vi "Dashboard Main.vi"() -> ()   [LabVIEW 2012]
uses:
  <vilib>/event_ctls.llb/eventvkey.ctl
  <vilib>/Utility/miscctls.llb/LVPointTypeDef.ctl
  <vilib>/Utility/config.llb/Read Key (String).vi
  <vilib>/Utility/config.llb/Read Key (I32).vi
  <vilib>/Utility/config.llb/Write Key (String).vi
  <vilib>/Utility/config.llb/Write Key (I32).vi
  <vilib>/Utility/config.llb/NI_LVConfig.lvlib
panel:
  out "Battery Value":dbl(slide) scale=0.0..14.0 scale format="%#_2e"
  out "Battery":sgl(graph)
  in  "Camera Settings":T1={"Frate Rate"=30, "Compression"=30, "Size"=0} {"Frate Rate" scale=1.0..30.0; "Size" items=["640x480", "320x240", "160x120"]}
  out "Mode":T2(ring)=enum.""
  out "Camera IP":string="10.16.76.11"
  out "JS1 Z":dbl(slide) scale=-1.0..1.0 scale format="%#_2e"
  out "JS2 Z":dbl(slide) scale=-1.0..1.0 scale format="%#_2e"
  out "Joystick 1":cluster{"X":dbl, "Y":dbl}[](graph)
  out "Joystick 2":cluster{"X":dbl, "Y":dbl}[](graph)
  out "JS Buttons 1":T3
  out "JS Buttons 2":T3
  out "MotorSlide4":dbl(slide) scale=-1.0..1.0 scale format="%#_2e"
  out "MotorSlide3":dbl(slide) scale=-1.0..1.0 scale format="%#_2e"
  out "MotorSlide2":dbl(slide) scale=-1.0..1.0 scale format="%#_2e"
  in  "MotorName3":string="Front Left"
  in  "MotorName4":string="Front Right"
  in  "MotorName1":string="Rear Left"
  in  "MotorName2":string="Rear Right"
  out "MotorChart4":dbl(graph)
  out "MotorChart3":dbl(graph)
  out "MotorChart2":dbl(graph)
  out "MotorSlide1":dbl(slide) scale=-1.0..1.0 scale format="%#_2e"
  out "MotorChart1":dbl(graph)
  out "Robot IP":string="0.0.0.0"
  in  "Dashboard Tab":enum32{"Operation", "Test", "Checklist"}(tab)
  out "Dashboard Code Verzion":string
  out "Robot Code Verzion":string
  out "Gyro":dbl
  out "Encoder Average":dbl
  out "Right Encoder":dbl
  out "Left Encoder":dbl
  out "Vision Angle":dbl
  in  "Slider":dbl(slide) scale=0.0..100.0 scale format="%#_3g"
  in  "On/Off":bool caption="Solenoid"
  in  "Test Name":u16(ring) items=["Select the test to run...", "Example Test", "-------------------------------", "List of tests is built in robot code.", "Replace with your own automated tests."]
  in  "Test Tree":string(tree)
  in  "Motor":cluster{"Value":dbl, "Enable":bool} {"Value" scale=-1.0..1.0 scale format="%#_3g"}
  out "Progress":T4 {"Test Progress" scale=0.0..100.0}
  in  "Rev/Fwd":cluster{"Forward":bool, "Reverse":bool}
  in  "Ring":u16(ring) items=["Auto", "Fixed indoor", "Fixed outdoor 1", "Fixed outdoor 2", "Fixed fluorescent 1", "Fixed fluorescent 2", "Hold current"]
  in  "Listbox":i32(listbox)
  in  "Viewer":T5(tab)
  out "Mbps":dbl format="%#.1g"
  in  "Enable":bool=TRUE
  in  "DB Camera Config":bool
  out "Mbps":bool
  out "fps":dbl format="%#.1g"
  out "Image Error Message":string="Timeout in Camera Communications"
  out "Camera Image":T6(plugin-control)
  out "Buttons 1":cluster{"1":bool, "2":bool, "3":bool}
  out "Kinect 1":cluster{"X":dbl, "Y":dbl, "Z":dbl} {"X" scale=1.0..-1.0; "Y" scale=1.0..-1.0; "Z" scale=1.0..-1.0}
  out "Buttons 2":cluster{"1":bool, "2":bool, "3":bool}
  out "Kinect 2":cluster{"X":dbl, "Y":dbl, "Z":dbl} {"X" scale=1.0..-1.0; "Y" scale=1.0..-1.0; "Z" scale=1.0..-1.0}
  out "Version":string
  out "Skeleton Picture":picture
  out "Players":i8
  out "Tree":string(tree)
  # "Drive & Motors"
  # "Robot IP:"
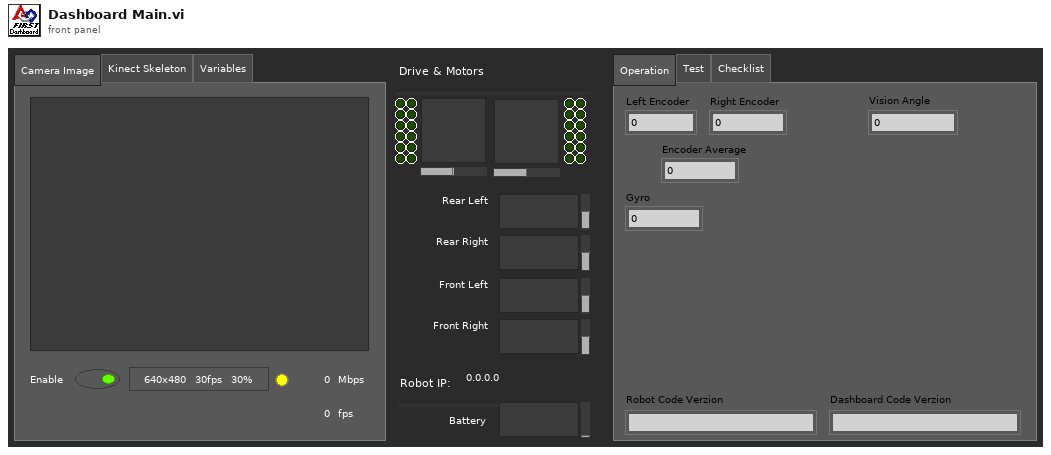
[diagram p1: front panel]
types:
  T1 = cluster{"Frate Rate":i32, "Compression":i32, "Size":u16}
  T2 = enum8{"Tele-Op Disabled", "Tele-Op Enabled", "Auto Disabled", "Auto Enabled", "Test Disabled", "Test Enabled", ""}
  T3 = cluster{bool, bool, bool, bool, bool, bool, bool, bool, bool, bool, bool, bool}
  T4 = cluster{"Test Progress":u8, "Test Progress Text":string}
  T5 = enum32{"Camera Image", "Kinect Skeleton", "Variables"}
  T6 = typedef "IMAQ Image.ctl" = refnum<image>
  T7 = typedef "Image Type" = u32
  T8 = cluster{"Competition mode":bool, "Robot Link":bool, "Autonomous":bool, "Enabled":bool, "E-Stop":bool, "Simulated":bool, "TestMode":bool, "Docked Window":bool}
  T9 = cluster{"Boolean Array[0]":bool, "Boolean Array[1]":bool, "Boolean Array[2]":bool, "Boolean Array[3]":bool, "Boolean Array[4]":bool, "Boolean Array[5]":bool, "Boolean Array[6]":bool, "Boolean Array[7]":bool, "Boolean Array[8]":bool, "Boolean Array[9]":bool, "Boolean Array[10]":bool, "Boolean Array[11]":bool}
  T10 = typedef "LVPointTypeDef.ctl" = cluster{"Horizontal":i16, "Vertical":i16}
  T11 = typedef "LVRectTypeDef.ctl" = cluster{"Left":i16, "Top":i16, "Right":i16, "Bottom":i16}
  T12 = typedef "LVBoundsTypeDef.ctl" = cluster{"Width":u32, "Height":u32}
  T13 = typedef "SkeletonTrackState.ctl" = enum32{"NotTracked", "PositionOnly", "Tracked"}
  T14 = cluster{"TrackingState":u8[], "Position":cluster{"x":sgl, "y":sgl, "z":sgl}, cluster{"x":sgl, "y":sgl, "z":sgl, sgl}[], "TrackState":T13}
  T15 = cluster{cluster{"ScaledToPercentRange":dbl, "ScaledToPercentRange":dbl, "ScaledToPercentRange":dbl}, cluster{bool, bool, bool}}[]
  T16 = cluster{cluster{"ScaledToPercentRange":dbl, "ScaledToPercentRange":dbl, "ScaledToPercentRange":dbl}, cluster{bool, bool, bool}}
  T17 = cluster{"ScaledToPercentRange":dbl, "ScaledToPercentRange":dbl, "ScaledToPercentRange":dbl}
  T18 = typedef "NI_LVConfig.lvlib/Config Data RefNum.ctl" = refnum<k1>
  T19 = typedef "eventvkey.ctl" = enum16{"ASCII", "Enter", "Return", "Shift", "Ctrl", "Alt", "Cmd", "Opt", "Caps", "NumLock", "Clear", "Break", "Up", "Down", "Left", "Right", "Insert", "Delete", "Home", "End", "PageUp", "PageDown", "Escape", "Help", "Pause", "ScrollLock", "F1", "F2", "F3", "F4", "F5", "F6", "F7", "F8", "F9", "F10", "F11", "F12", "F13", "F14", "F15", "F16", "F17", "F18", "F19", "F20", "F21", "F22", "F23", "F24", "Play", "VolumeUp", "VolumeDown", "Mute", "Two Byte Char"}
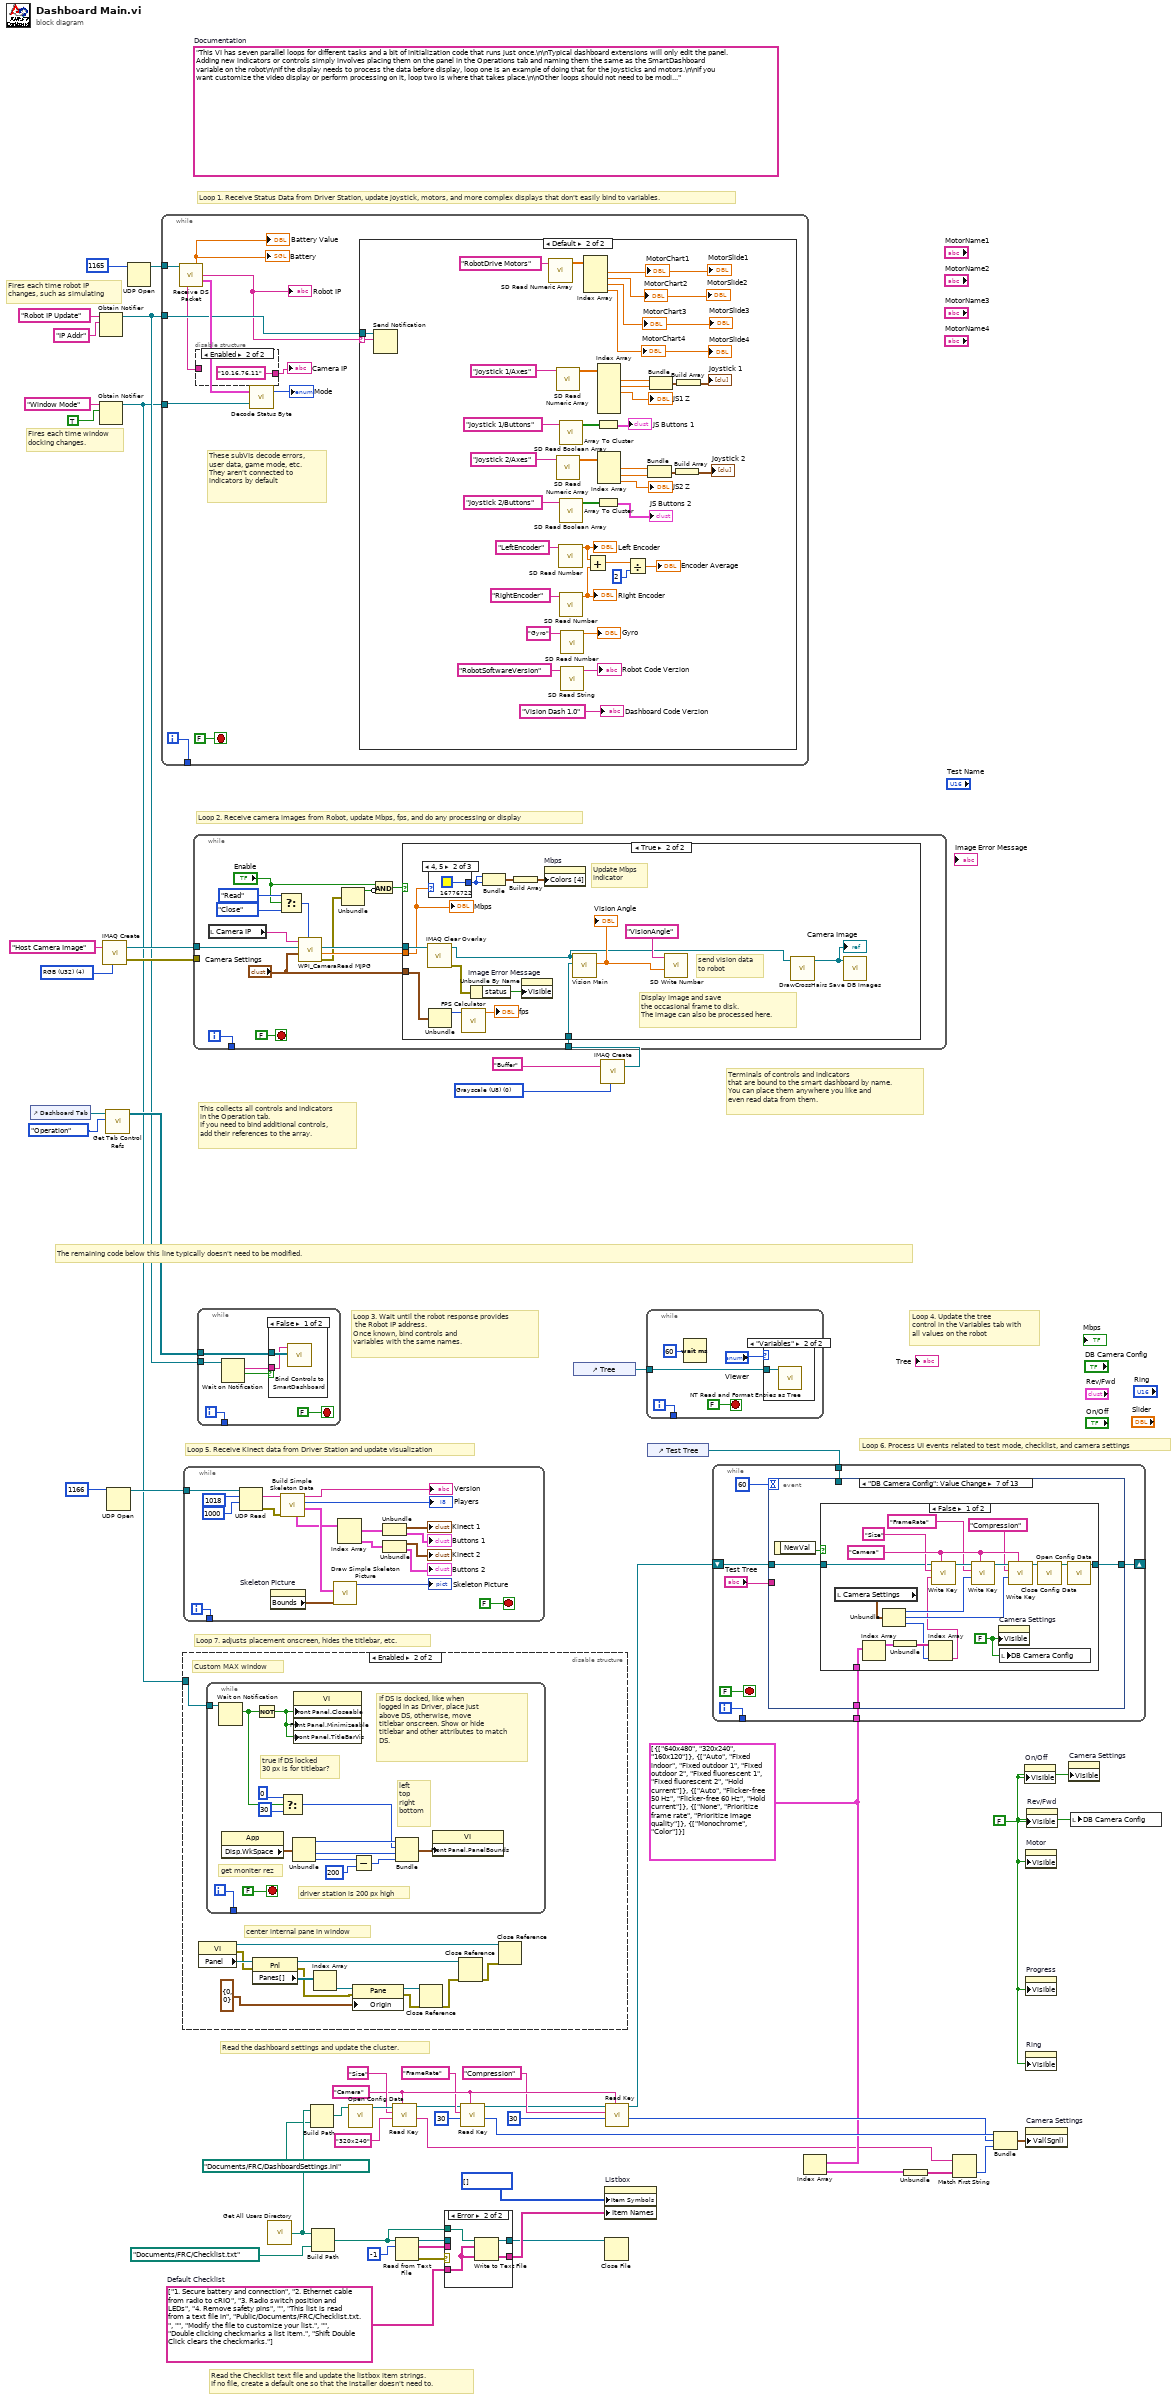
[diagram p0: block diagram]
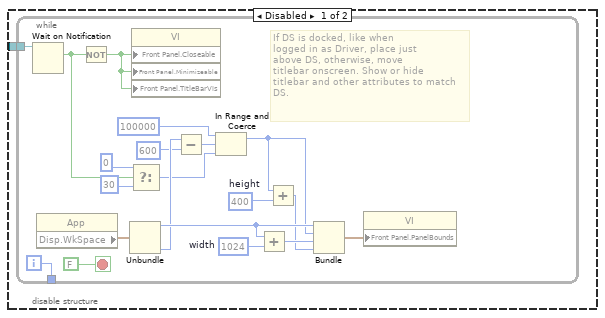
[diagram p2: hidden frame]
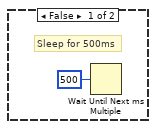
[diagram p4: hidden frame]
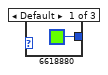
[diagram p5: hidden frame]
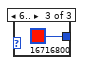
[diagram p6: hidden frame]
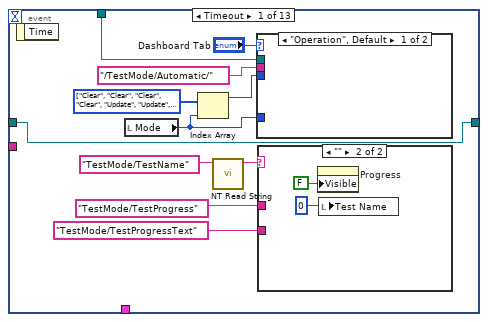
[diagram p8: hidden frame]
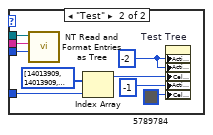
[diagram p9: hidden frame]
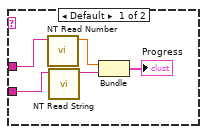
[diagram p10: hidden frame]
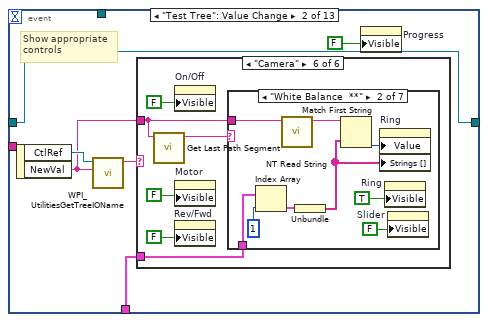
[diagram p11: hidden frame]
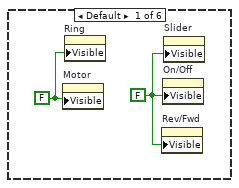
[diagram p12: hidden frame]
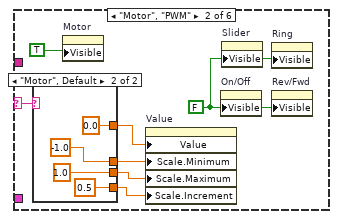
[diagram p13: hidden frame]
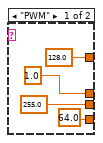
[diagram p14: hidden frame]
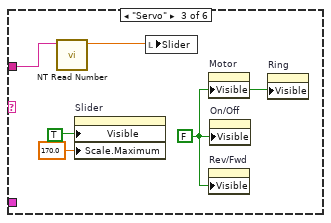
[diagram p15: hidden frame]
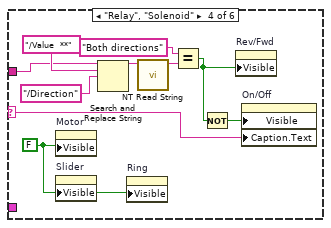
[diagram p16: hidden frame]
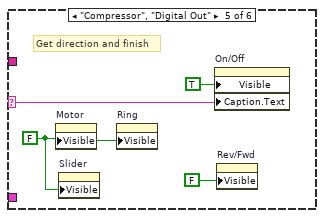
[diagram p17: hidden frame]
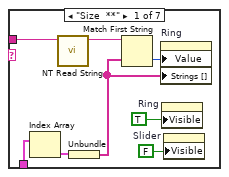
[diagram p18: hidden frame]
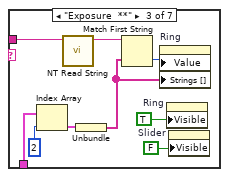
[diagram p19: hidden frame]
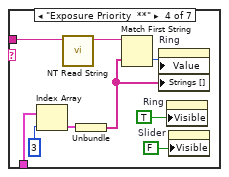
[diagram p20: hidden frame]
diagram:
  w2 = T7 0 items=["Grayscale (U8)", "Grayscale (I16)", "Grayscale (SGL)", "Complex (CSG)", "RGB (U32)", "HSL (U32)", "RGB (U64)", "Grayscale (U16)"] ("Image Type")
  w24 = "Camera"
  w16 = cluster{string[]}[] [{["640x480", "320x240", "160x120"]}, {["Auto", "Fixed indoor", "Fixed outdoor 1", "Fixed outdoor 2", "Fixed fluorescent 1", "Fixed fluorescent 2", "Hold current"]}, {["Auto", "Flicker-free 50 Hz", "Flicker-free 60 Hz", "Hold current"]}, {["None", "Prioritize frame rate", "Prioritize image quality"]}, {["Monochrome", "Color"]}]
  w32 = string[] ["1. Secure battery and connection", "2. Ethernet cable from radio to cRIO", "3. Radio switch position and LEDs", "4. Remove safety pins", "", "This list is read from a text file in", "Public/Documents/FRC/Checklist.txt.", "", "Modify the file to customize your list.", "", "Double clicking checkmarks a list item.", "Shift Double Click clears the checkmarks."]  # Default Checklist
  w30 = FALSE ("Visible")
  (unwired) "This VI has seven parallel loops for different tasks and a bit of initialization code that runs just once.\n\nTypical dashboard extensions will only edit the panel. Adding new indicators or controls simply involves placing them on the panel in the Operations tab and naming them the same as the SmartDashboard variable on the robot\n\nIf the display needs to process the data before display, loop one is an example of doing that for the joysticks and motors.\n\nIf you want customize the video display or perform processing on it, loop two is where that takes place.\n\nOther loops should not need to be modified. They are pretty standard, and document the task they perform."  # Documentation
  w53 = T7 4 items=["Grayscale (U8)", "Grayscale (I16)", "Grayscale (SGL)", "Complex (CSG)", "RGB (U32)", "HSL (U32)", "RGB (U64)"] ("Image Type")
  # "Fires each time robot IP\nchanges, such as simulating"
  # "Fires each time window\ndocking changes."
  # "Read the Checklist text file and update the listbox item strings.\nIf no file, create a default one so that the installer doesn't need to."
  # "This collects all controls and indicators\nin the Operation tab.\nIf you need to bind additional controls,\nadd their references to the array."
  # "The remaining code below this line typically doesn't need to be modified."
  # "Loop 6. Process UI events related to test mode, checklist, and camera settings"
  # "Read the dashboard settings and update the cluster."
  # "Terminals of controls and indicators\nthat are bound to the smart dashboard by name.\nYou can place them anywhere you like and\neven read data from them."
  # "Loop 4. Update the tree\ncontrol in the Variables tab with\nall values on the robot"
  # "Loop 3. Wait until the robot response provides\n the Robot IP address.\nOnce known, bind controls and\nvariables with the same names."
  # "Loop 5. Receive Kinect data from Driver Station and update visualization"
  # "Loop 7. adjusts placement onscreen, hides the titlebar, etc."
  # "Loop 1. Receive Status Data from Driver Station, update joystick, motors, and more complex displays that don't easily bind to variables."
  # "Loop 2. Receive camera images from Robot, update Mbps, fps, and do any processing or display"
  n1 = control-ref of="Dashboard Tab"() -> (w46:refnum<vi>)
  n2 = Obtain Notifier(name (unnamed)="Robot IP Update", notification data type="IP Addr" ("name (unnamed)")) -> (notifier out=w43:refnum<notifier>)  [unwired: 2 in, 2 out]
  n3 = Obtain Notifier(name (unnamed)="Window Mode", notification data type=TRUE) -> (notifier out=w36:refnum<notifier>)  [unwired: 2 in, 2 out]
  n4 = call "IMAQ Create"("Image Name"="Host Camera Image", "Image Type"=w53) -> ("New Image"=w51:T6, "error out"=w50:errorcluster)  [unwired: 2 in, 1 out]
  n5 = call <vilib>:"Get Tab Control Refs.vi"("Page Index"=enum32{"Operation", "Test"}."Operation" ("Dashboard Tab"), "TabControl in"=w46) -> ("ControlsOnPage"=w47:refnum<vi>[])  [unwired: 9 in]
  n6 = UDP Open(11:u16 1166 ("port")) -> (port=w48:refnum<k16>)  [unwired: 2 in, 4 out]
  n7 = UDP Open(11:u16 1165 ("port")) -> (port=w54:refnum<k16>)  [unwired: 2 in, 4 out]
  n8 = while {
    tunnel: w54 -> [w64]
    tunnel: w43 -> [w59]
    tunnel: w36 -> [w62]
    tunnel: [w60] -> _
    i -> [w60]
    stop <- FALSE stop-if-true
    # "These subVIs decode errors, user data, game mode, etc.\nThey aren't connected to indicators by default"
    n9 = call "Receive DS Packet.vi"("Recv Socket"=w64) -> ("Battery"=→"Battery" →"Battery Value":sgl, "Robot IP Address"=w58:string, "Status"=w65:T8, "Camera IP Address"=w56:string)  [unwired: 1 in, 10 out]
    "Robot IP" <- w58
    n10 = disable-structure shown="Enabled" {
      disable-tunnel: [w67 "10.16.76.11" ("Camera IP")] -> w57
      disable-tunnel: w56 -> [w67 _]
      frame Disabled {
      }
      frame Enabled {
      }
    }
    "Camera IP" <- w57
    n11 = call "Decode Status Byte.vi"("Window Mode Notifier"=w62, "Status"=w65) -> ("Mode"=→"Mode":T2)  [unwired: 1 out]
    n12 = case shown="Default" w58 {
      selector: w58 -> [_ w81]
      tunnel: w59 -> [_ w82]
      frame "0.0.0.0" {
        # "Robot not responding, don't poll the variables"
      }
      frame Default {
        n13 = Send Notification(notification=w81, notifier=w82) -> ()  [unwired: 1 in, 2 out]
        n14 = call <vilib>:"SD Read Numeric Array.vi"("Name"="RobotDrive Motors") -> ("Numeric Array"=w105:dbl[])  [unwired: 8 in, 2 out]
        n15 = call <vilib>:"SD Read Numeric Array.vi"("Name"="Joystick 1/Axes") -> ("Numeric Array"=w98:dbl[])  [unwired: 8 in, 2 out]
        n16 = call <vilib>:"SD Read Numeric Array.vi"("Name"="Joystick 2/Axes") -> ("Numeric Array"=w92:dbl[])  [unwired: 8 in, 2 out]
        n17 = call <vilib>:"SD Read Number.vi"("Name"="LeftEncoder") -> ("Numeric"=w77:dbl)  [unwired: 8 in, 2 out]
        "Left Encoder" <- w77
        n18 = call <vilib>:"SD Read Boolean Array.vi"("Name"="Joystick 1/Buttons") -> ("Boolean Array"=w100:bool[])  [unwired: 8 in, 2 out]
        n19 = call <vilib>:"SD Read Boolean Array.vi"("Name"="Joystick 2/Buttons") -> ("Boolean Array"=w91:bool[])  [unwired: 8 in, 2 out]
        n20 = call <vilib>:"SD Read Number.vi"("Name"="RightEncoder") -> ("Numeric"=w76:dbl)  [unwired: 8 in, 2 out]
        "Right Encoder" <- w76
        n21 = call <vilib>:"SD Read Number.vi"("Name"="Gyro") -> ("Numeric"=→"Gyro":dbl)  [unwired: 8 in, 2 out]
        n22 = call <vilib>:"SD Read String.vi"("Name"="RobotSoftwareVersion") -> ("String"=→"Robot Code Verzion":string)  [unwired: 8 in, 2 out]
        n23 = Index Array(array=w105) -> (element #1=→"MotorChart1" →"MotorSlide1":dbl, element #2=→"MotorSlide2" →"MotorChart2":dbl, element #3=→"MotorChart3" →"MotorSlide3":dbl, element #4=→"MotorChart4" →"MotorSlide4":dbl)  [unwired: 4 in]
        n24 = Add(x=w77, y=w76) -> (x+y=w74:dbl)
        n25 = Array To Cluster(array=w100) -> (cluster=→"JS Buttons 1":T9)
        n26 = Array To Cluster(array=w91) -> (cluster=→"JS Buttons 2":T9)
        n27 = Index Array(array=w98) -> (element #1=w95:dbl, element #2=w96:dbl, element #3=→"JS1 Z":dbl)  [unwired: 6 in, 3 out]
        n28 = Index Array(array=w92) -> (element #1=w87:dbl, element #2=w86:dbl, element #3=→"JS2 Z":dbl)  [unwired: 3 in]
        n29 = Divide(x=w74, y=2) -> (x/y=→"Encoder Average":dbl)
        n30 = Bundle("Numeric"=w87, "Numeric"=w86) -> (w88:cluster{"Numeric":dbl, "Numeric":dbl})  [unwired: 1 in]
        n31 = Bundle("Numeric"=w95, "Numeric"=w96) -> (w94:cluster{"Numeric":dbl, "Numeric":dbl})  [unwired: 1 in]
        n32 = Build Array(w88) -> (→"Joystick 2":cluster{"Numeric":dbl, "Numeric":dbl}[])
        n33 = Build Array(w94) -> (→"Joystick 1":cluster{"Numeric":dbl, "Numeric":dbl}[])
        "Dashboard Code Verzion" <- "Vision Dash 1.0" ("Dashboard Code Verzion")
      }
    }
  }
  n34 = disable-structure shown="Enabled" {
    disable-tunnel: w36 -> [w109 w142]
    frame Disabled {
      n35 = while {
        tunnel: w109 -> [w128]
        tunnel: [w126] -> _
        i -> [w126]
        stop <- FALSE stop-if-true
        w118 = 1024  # width
        w121 = 400  # height
        # "If DS is docked, like when\nlogged in as Driver, place just\nabove DS, otherwise, move\ntitlebar onscreen. Show or hide\ntitlebar and other attributes to match\nDS."
        n36 = Wait on Notification(notifier=w128) -> (notification=w113:bool)  [unwired: 3 in, 3 out]
        n37 = property class="App"() -> ("Disp.WkSpace"=w124:T11)  [unwired: 2 in, 2 out]
        n38 = Not(x=w113) -> (.not. x?=w127:bool)
        n39 = Unbundle(w124) -> ("Left"=w122:i16, "Bottom"=w119:i16)  [unwired: 2 out]
        n40 = Select(t=0, s=w113, f=30) -> (s? t:f=w112:i32)
        n41 = property class="VI"("Front Panel.Closeable"=w127, "Front Panel.Minimizeable"=w127, "Front Panel.TitleBarVis"=w127) -> ()  [unwired: 2 in, 2 out]
        n42 = Subtract(x=w119, y=600) -> (x-y=w116:i32)
        n43 = In Range and Coerce(upper limit=100000, x=w116, lower limit=w112) -> (coerced(x)=w110:i32)  [unwired: 1 out]
        n44 = Add(x=w122, y=w118) -> (x+y=w123:i32)
        n45 = Add(x=w110, y=w121) -> (x+y=w120:i32)
        n46 = Bundle("Left"=w122, w110, w123, w120) -> (w125:cluster{"Left":i16, i32, i32, i32})  [unwired: 1 out]
        n47 = property class="VI"("Front Panel.PanelBounds"=w125) -> ()  [unwired: 2 in, 2 out]
      }
    }
    frame Enabled {
      # "center internal pane in window"
      # "Custom MAX window"
      n48 = property class="VI"() -> (reference out=w135:refnum<vi>, error out=w134:errorcluster, "Panel"=w141:refnum<vi>)  [unwired: 2 in]
      n49 = while {
        tunnel: w142 -> [w156]
        tunnel: [w154] -> _
        i -> [w154]
        stop <- FALSE stop-if-true
        # "driver station is 200 px high"
        # "true if DS locked\n30 px is for titlebar?"
        # "left\ntop\nright\nbottom"
        # "get moniter rez"
        # "If DS is docked, like when\nlogged in as Driver, place just\nabove DS, otherwise, move\ntitlebar onscreen. Show or hide\ntitlebar and other attributes to match\nDS."
        n50 = Wait on Notification(notifier=w156) -> (notification=w148:bool)  [unwired: 3 in, 3 out]
        n51 = property class="App"() -> ("Disp.WkSpace"=w152:T11)  [unwired: 2 in, 2 out]
        n52 = Not(x=w148) -> (.not. x?=w155:bool)
        n53 = Select(t=0, s=w148, f=30) -> (s? t:f=w146:i32)
        n54 = Unbundle(w152) -> ("Left"=w151:i16, "Right"=w147:i16, "Bottom"=w144:i16)  [unwired: 1 out]
        n55 = property class="VI"("Front Panel.Closeable"=w155, "Front Panel.Minimizeable"=w155, "Front Panel.TitleBarVis"=w155) -> ()  [unwired: 2 in, 2 out]
        n56 = Subtract(x=w144, y=i16 200) -> (x-y=w145:i16)
        n57 = Bundle("Left"=w151, w146, "Right"=w147, w145) -> (w153:cluster{"Left":i16, i32, "Right":i16, i16})  [unwired: 1 out]
        n58 = property class="VI"("Front Panel.PanelBounds"=w153) -> ()  [unwired: 2 in, 2 out]
      }
      n59 = property class="Pnl"(reference=w141, error in=w134) -> (reference out=w136:refnum<vi>, error out=w133:errorcluster, "Panes[]"=w140:refnum<vi>[])
      n60 = Index Array(array=w140) -> (element=w139:refnum<vi>)  [unwired: 1 in]
      n61 = property class="Pane"(reference=w139, error in=w133, "Origin"=T10 {"Horizontal"=0, "Vertical"=0}) -> (reference out=w137:refnum<vi>, error out=w132:errorcluster)
      n62 = Close Reference(reference=w137, error in (no error)=w132) -> (error out=w131:errorcluster)
      n63 = Close Reference(reference=w136, error in (no error)=w131) -> (error out=w130:errorcluster)
      n64 = Close Reference(reference=w135, error in (no error)=w130) -> ()  [unwired: 1 out]
    }
  }
  n65 = while {
    tunnel: w48 -> [w174]
    tunnel: [w159] -> _
    i -> [w159]
    stop <- FALSE stop-if-true
    n66 = UDP Read(connection ID=w174, max size (548)=1018 ("bytes to read"), timeout ms (25000)=1000) -> (data out=w168:string, error out=w158:errorcluster)  [unwired: 1 in, 3 out]
    n67 = property on="Skeleton Picture" class="Pict"() -> ("Bounds"=w170:T12)  [unwired: 2 in, 2 out]
    n68 = call "Build Simple Skeleton Data.vi"("error in (no error)"=w158, "data in"=w168) -> ("Skeleton Data"=w169:T14, "NumPlayers"=→"Players":i8, "Version String"=→"Version":string, "Simple Joystick Info"=w166:T15)  [unwired: 5 in, 1 out]
    n69 = call "Draw Simple Skeleton Picture.vi"("Bounds"=w170, "Simple Skeleton"=w169) -> ("new picture out"=→"Skeleton Picture":picture)  [unwired: 9 in]
    n70 = Index Array(array=w166) -> (element #1=w165:T16, element #2=w164:T16)  [unwired: 2 in]
    n71 = Unbundle(w165) -> (→"Kinect 1":T17, →"Buttons 1":cluster{bool, bool, bool})
    n72 = Unbundle(w164) -> (→"Kinect 2":T17, →"Buttons 2":cluster{bool, bool, bool})
  }
  n73 = while {
    tunnel: w47 -> [w182]
    tunnel: w43 -> [w179]
    tunnel: [w177] -> _
    i -> [w177]
    stop <- FALSE stop-if-true
    n74 = Wait on Notification(notifier=w179) -> (notification=w178:string, timed out?=w180:bool)  [unwired: 3 in, 2 out]
    n75 = case shown="False" w180 {
      tunnel: w182 -> [w184 _]
      tunnel: w178 -> [w183 _]
      frame False {
        n76 = call <vilib>:"Bind Controls to SmartDashboard.vi"("Bound Control Refs"=w184, "Server IP Address"=w183) -> ()  [unwired: 10 in]
      }
      frame True {
      }
    }
  }
  n77 = call "Get All Users Directory.vi"() -> ("All User Path"=w29:path)
  n78 = Build Path(base path=w29, name or relative path=path "Documents/FRC/DashboardSettings.ini") -> (appended path=w28:path)
  n79 = Build Path(base path=w29, name or relative path=path "Documents/FRC/Checklist.txt") -> (appended path=w33:path)
  n80 = call <vilib>:"Open Config Data.vi"("configuration file path"=w28) -> ("refnum"=w27:T18)  [unwired: 8 in, 2 out]
  n81 = call-poly <vilib>:"Read Key.vi"("section"=w24, "default value"="320x240", "key"="Size", "refnum"=w27) -> ("value"=w14:string, "refnum out"=w9:T18)  [unwired: 2 in, 4 out]
  n82 = Read from Text File(file (use dialog)=w33, count=-1 ("timeout ms (25000)")) -> (refnum out=w11:refnum<file>, text=w34:string[], error out=w35:errorcluster)  [unwired: 2 in, 1 out]
  n83 = case shown="Error" w35 {
    tunnel: w34 -> [w186 _]
    tunnel: [w186 w188] -> w31
    tunnel: w32 -> [_ w188]
    tunnel: w33 -> [_ w189]
    tunnel: [w185 w187] -> w10
    tunnel: w11 -> [w185 _]
    frame No Error {
    }
    frame Error {
      n84 = Write to Text File(file (use dialog)=w189, text=w188) -> (refnum out=w187:refnum<file>)  [unwired: 2 in, 2 out]
    }
  }
  n85 = call-poly <vilib>:"Read Key.vi"("section"=w24, "default value"=30, "key"="FrameRate", "refnum"=w9) -> ("value"=w19:i32, "refnum out"=w8:T18)  [unwired: 1 in, 5 out]
  n86 = control-ref of="Tree"() -> (w5:refnum<vi>)
  n87 = call "IMAQ Create"("Image Name"="Buffer", "Image Type"=w2) -> ("New Image"=w1:T6)  [unwired: 3 in, 1 out]
  n88 = while {
    tunnel: w51 -> [w200]
    tunnel: w50 -> [_]
    tunnel: [w203] -> _
    tunnel: w1 -> [w190]
    i -> [w203]
    stop <- FALSE stop-if-true
    n89 = local read "Camera IP"() -> (w202:string)
    n90 = Select(t=enum16{"Read", "Reopen", "Close"}."Read" ("Operation"), s="Enable", f=enum16{"Read", "Reopen", "Close"}."Close" ("Operation")) -> (s? t:f=w195:enum16{"Read", "Reopen", "Close"})
    n91 = call <vilib>:"WPI_CameraRead MJPG.vi"("Operation"=w195, "Camera Settings"="Camera Settings", "Image"=w200, "address"=w202) -> ("error out"=w194:errorcluster, "Bandwidth (kbps)"=w198:dbl, "Image Out"=w199:T6)  [unwired: 5 in]
    n92 = Unbundle(w194) -> ("status"=w192:bool)  [unwired: 2 out]
    n93 = Compound Arithmetic op=AND("Enable", invert w192) -> (w191:bool)
    n94 = case shown="True" w191 {
      tunnel: "Camera Settings" -> [_ w212]
      tunnel: w199 -> [_ w215]
      tunnel: w198 -> [_ w214]
      tunnel: w190 -> [_ w210]
      frame False {
        # "Sleep for 500ms"
        n95 = Wait Until Next ms Multiple(millisecond multiple=u32 500) -> ()  [unwired: 1 out]
      }
      frame True {
        # "send vision data\nto robot"
        # "Display image and save\nthe occasional frame to disk.\nThe image can also be processed here."
        # "Update Mbps\nindicator"
        n96 = call "IMAQ Clear Overlay"("Image"=w215) -> ("error out"=w219:errorcluster, "Image Out"=w206:T6)  [unwired: 2 in, 7 out]
        n97 = case shown="4, 5" w214 {
          tunnel: [u32 6618880 ("Color Box") u32 16776722 ("Color Box") u32 16716800 ("Color Box")] -> w216
          frame Default {
          }
          frame 4, 5 {
          }
          frame 6.. {
          }
        }
        n98 = Unbundle(w212) -> ("Frate Rate"=w211:i32)  [unwired: 2 out]
        n99 = call "FPS Calculator.vi"("Average Count"=w211) -> ("fps"=→"fps":dbl)  [unwired: 10 in]
        n100 = Unbundle By Name(w219) -> ("status"=w220:bool)
        n101 = Bundle("Color Box"=w216, "Color Box"=w216) -> (w218:cluster{"Color Box":u32, "Color Box":u32})  [unwired: 1 out]
        n102 = Build Array(w218) -> (w217:cluster{"Color Box":u32, "Color Box":u32}[])
        n103 = property on="Image Error Message" class="Str"("Visible"=w220) -> ()  [unwired: 2 in, 2 out]
        n104 = property on="Mbps" class="Bool (strict)"("Colors [4]"=w217) -> ()  [unwired: 2 in, 2 out]
        n105 = call "Vision Main.vi"("Frame Buffer"=w210, "Camera Image"=w206) -> ("Chosen Target Angle"=w208:dbl)  [unwired: 8 in, 1 out]
        "Vision Angle" <- w208
        n106 = call <vilib>:"SD Write Number.vi"("Numeric"=w208, "Name"="VisionAngle") -> ()  [unwired: 8 in, 2 out]
        n107 = call "DrawCrossHairs.vi"("Image In"=w206) -> ("Image Out"=w207:T6)  [unwired: 10 in]
        "Camera Image" <- w207
        n108 = call "Save DB Images.vi"("Image"=w207) -> ()  [unwired: 2 in, 1 out]
        "Mbps" <- w214
      }
    }
  }
  n109 = property on="Listbox" class="LstBox (strict)"("Item Symbols"=i32[] [], "Item Names"=w31) -> ()  [unwired: 2 in, 2 out]
  n110 = Close File(refnum=w10) -> ()  [unwired: 1 in, 2 out]
  n111 = call-poly <vilib>:"Read Key.vi"("section"=w24, "default value"=30, "key"="Compression", "refnum"=w8) -> ("value"=w18:i32, "refnum out"=w6:T18)  [unwired: 1 in, 5 out]
  n112 = while {
    tunnel: [w225] -> _
    tunnel: w5 -> [w224]
    i -> [w225]
    stop <- FALSE stop-if-true
    n113 = Wait (ms)(milliseconds to wait=u32 60) -> ()  [unwired: 1 out]
    n114 = case shown="\"Variables\"" "Viewer" {
      tunnel: w224 -> [_ w229]
      frame Default {
      }
      frame "Variables" {
        n115 = call <vilib>:"NT Read and Format Entries as Tree.vi"("Tree Refnum"=w229) -> ()  [unwired: 9 in, 2 out]
      }
    }
  }
  n116 = control-ref of="Test Tree"() -> (w4:refnum<vi>)
  n117 = while {
    tunnel: w16 -> [w234]
    shift-right: [w233] -> _
    shift-left: w6 -> [w232]
    tunnel: [w231] -> _
    tunnel: w4 -> [w230]
    i -> [w231]
    stop <- FALSE stop-if-true
    n118 = event shown="[6] \"DB Camera Config\": Value Change" {
      selector: _ -> [_ _ _ _ _ _ _ _ _ _ _ _ _]
      dyn-events: _ -> [_ _ _ _ _ _ _ _ _ _ _ _ _]
      timeout: u32 60 ("milliseconds to wait") -> [_ _ _ _ _ _ _ _ _ _ _ _ _]
      tunnel: w230 -> [w244 _ _ _ _ _ _ _ _ _ _ _ _]
      tunnel: "Test Tree" -> [_ _ _ _ _ _ _ _ w438 w446 w448 w452 w460]
      tunnel: w234 -> [_ w266 _ _ _ _ w402 w432 _ _ _ _ _]
      tunnel: [w238 w265 _ w368 w376 w388 w401 w425 w437 w444 w447 w451 w459] -> w233
      tunnel: w232 -> [w238 w265 _ w368 w376 w388 w400 w425 w437 w444 w447 w451 w459]
      event Timeout {
        w243 = enum16{"Update", "Clear"}[] [enum."Clear", enum."Clear", enum."Clear", enum."Clear", enum."Update", enum."Update", enum."Clear"] items=["Update", "Clear"]
        n119 = event-data() -> ()  [unwired: 1 in, 1 out]
        n120 = local read "Mode"() -> (w241:T2)
        n121 = Index Array(array=w243, index=w241) -> (element=w242:enum16{"Update", "Clear"})
        n122 = call <vilib>:"NT Read String.vi"("Name"="TestMode/TestName") -> ("String"=w247:string)  [unwired: 9 in, 1 out]
        n123 = case shown="\"Operation\", Default" "Dashboard Tab" {
          tunnel: w244 -> [_ w257]
          tunnel: "/TestMode/Automatic/" ("Name Pattern") -> [_ w256]
          tunnel: w242 -> [_ w255]
          tunnel: w241 -> [_ w253]
          frame "Operation", Default {
          }
          frame "Test" {
            w252 = -2 ("Active Item:Row Number")
            n124 = call <vilib>:"NT Read and Format Entries as Tree.vi"("Operation"=w255, "Name Pattern"=w256, "Tree Refnum"=w257) -> ()  [unwired: 7 in, 2 out]
            n125 = Index Array(array=u32[] [14013909, 14013909, 14013909, 14013909, 14013909, 16777215, 14013909], index=w253) -> (element=w251:u32)
            n126 = property on="Test Tree" class="Tree (strict)"("Active Item Row Number"=w252, "ActiveColNum"=w252, "CellBG"=w251, "Active Item Row Number"=-1 ("Active Item:Row Number"), "CellBG"=u32 5789784 ("Color Box")) -> ()  [unwired: 2 in, 2 out]
          }
        }
        n127 = case shown="\"\"" w247 {
          tunnel: "TestMode/TestProgress" ("Name") -> [w259 _]
          tunnel: "TestMode/TestProgressText" ("Name") -> [w258 _]
          frame Default {
            n128 = call <vilib>:"NT Read Number.vi"("Name"=w259) -> ("Numeric"=w260:dbl)  [unwired: 9 in, 1 out]
            n129 = call <vilib>:"NT Read String.vi"("Name"=w258) -> ("String"=w261:string)  [unwired: 9 in, 1 out]
            n130 = Bundle("Numeric"=w260, "String"=w261) -> (→"Progress":cluster{"Numeric":dbl, "String":string})  [unwired: 1 in]
          }
          frame "" {
            n131 = property on="Progress" class="Clust (strict)"("Visible"=FALSE) -> ()  [unwired: 2 in, 2 out]
            n132 = local write "Test Name"(u16 0) -> ()
          }
        }
      }
      event "Test Tree": Value Change {
        # "Show appropriate\ncontrols"
        n133 = event-data() -> ("CtlRef"=w269:refnum<vi>, "NewVal"=w267:string)  [unwired: 1 in]
        n134 = call <vilib>:"WPI_UtilitiesGetTreeIOName.vi"("NewVal"=w267, "TreeControl in"=w269) -> ("I/O Name"=w270:string)  [unwired: 9 in]
        n135 = case shown="\"Camera\"" w270 {
          selector: w270 -> [_ w277 _ w295 w304 _]
          tunnel: w267 -> [_ _ w292 w294 _ w311]
          tunnel: w266 -> [_ _ _ _ _ w310]
          frame Default {
            w272 = FALSE ("Visible")
            w271 = FALSE ("Visible")
            n136 = property on="Motor" class="Clust (strict)"("Visible"=w271) -> ()  [unwired: 2 in, 2 out]
            n137 = property on="Ring" class="Ring (strict)"("Visible"=w271) -> ()  [unwired: 2 in, 2 out]
            n138 = property on="Rev/Fwd" class="Clust (strict)"("Visible"=w272) -> ()  [unwired: 2 in, 2 out]
            n139 = property on="On/Off" class="Bool (strict)"("Visible"=w272) -> ()  [unwired: 2 in, 2 out]
            n140 = property on="Slider" class="Slide (strict)"("Visible"=w272) -> ()  [unwired: 2 in, 2 out]
          }
          frame "Motor", "PWM" {
            w278 = FALSE ("Visible")
            n141 = case shown="\"Motor\", Default" w277 {
              tunnel: [1.0 ("Value") -1.0 ("Value")] -> w276
              tunnel: [255.0 ("Value") 1.0 ("Value")] -> w275
              tunnel: [128.0 ("Value") 0.0 ("Value")] -> w274
              tunnel: [64.0 ("Value") 0.5 ("Value")] -> w273
              frame "PWM" {
              }
              frame "Motor", Default {
              }
            }
            n142 = property on="Motor" class="Clust (strict)"("Visible"=TRUE) -> ()  [unwired: 2 in, 2 out]
            n143 = property on="Value" class="Slide (strict)"("Value"=w274, "Scale.Minimum"=w276, "Scale.Maximum"=w275, "Scale.Increment"=w273) -> ()  [unwired: 2 in, 2 out]
            n144 = property on="On/Off" class="Bool (strict)"("Visible"=w278) -> ()  [unwired: 2 in, 2 out]
            n145 = property on="Slider" class="Slide (strict)"("Visible"=w278) -> ()  [unwired: 2 in, 2 out]
            n146 = property on="Ring" class="Ring (strict)"("Visible"=w278) -> ()  [unwired: 2 in, 2 out]
            n147 = property on="Rev/Fwd" class="Clust (strict)"("Visible"=w278) -> ()  [unwired: 2 in, 2 out]
          }
          frame "Servo" {
            w290 = FALSE ("Visible")
            n148 = call <vilib>:"NT Read Number.vi"("Name"=w292) -> ("Numeric"=w291:dbl)  [unwired: 9 in, 1 out]
            n149 = property on="Slider" class="Slide (strict)"("Visible"=TRUE, "Scale.Maximum"=170.0 ("Scale.Range:Maximum")) -> ()  [unwired: 2 in, 2 out]
            n150 = local write "Slider"(w291) -> ()
            n151 = property on="Motor" class="Clust (strict)"("Visible"=w290) -> ()  [unwired: 2 in, 2 out]
            n152 = property on="Rev/Fwd" class="Clust (strict)"("Visible"=w290) -> ()  [unwired: 2 in, 2 out]
            n153 = property on="On/Off" class="Bool (strict)"("Visible"=w290) -> ()  [unwired: 2 in, 2 out]
            n154 = property on="Ring" class="Ring (strict)"("Visible"=w290) -> ()  [unwired: 2 in, 2 out]
          }
          frame "Relay", "Solenoid" {
            w293 = FALSE ("Visible")
            n155 = property on="Motor" class="Clust (strict)"("Visible"=w293) -> ()  [unwired: 2 in, 2 out]
            n156 = property on="Slider" class="Slide (strict)"("Visible"=w293) -> ()  [unwired: 2 in, 2 out]
            n157 = Search and Replace String(input string=w294, search string="/Value  **", replace string="/Direction") -> (result string=w300:string)  [unwired: 5 in, 3 out]
            n158 = property on="Ring" class="Ring (strict)"("Visible"=w293) -> ()  [unwired: 2 in, 2 out]
            n159 = call <vilib>:"NT Read String.vi"("Name"=w300) -> ("String"=w298:string)  [unwired: 9 in, 1 out]
            n160 = Equal?(x="Both directions", y=w298) -> (x = y?=w296:bool)
            n161 = Not(x=w296) -> (.not. x?=w297:bool)
            n162 = property on="Rev/Fwd" class="Clust (strict)"("Visible"=w296) -> ()  [unwired: 2 in, 2 out]
            n163 = property on="On/Off" class="Bool (strict)"("Visible"=w297, "Caption.Text"=w295) -> ()  [unwired: 2 in, 2 out]
          }
          frame "Compressor", "Digital Out" {
            w303 = FALSE ("Visible")
            # "Get direction and finish"
            n164 = property on="Motor" class="Clust (strict)"("Visible"=w303) -> ()  [unwired: 2 in, 2 out]
            n165 = property on="Slider" class="Slide (strict)"("Visible"=w303) -> ()  [unwired: 2 in, 2 out]
            n166 = property on="Ring" class="Ring (strict)"("Visible"=w303) -> ()  [unwired: 2 in, 2 out]
            n167 = property on="On/Off" class="Bool (strict)"("Visible"=TRUE, "Caption.Text"=w304) -> ()  [unwired: 2 in, 2 out]
            n168 = property on="Rev/Fwd" class="Clust (strict)"("Visible"=FALSE) -> ()  [unwired: 2 in, 2 out]
          }
          frame "Camera" {
            n169 = call <vilib>:"Get Last Path Segment.vi"("String in"=w311) -> ("String out"=w312:string)  [unwired: 10 in]
            n170 = property on="On/Off" class="Bool (strict)"("Visible"=FALSE) -> ()  [unwired: 2 in, 2 out]
            n171 = property on="Motor" class="Clust (strict)"("Visible"=FALSE) -> ()  [unwired: 2 in, 2 out]
            n172 = property on="Rev/Fwd" class="Clust (strict)"("Visible"=FALSE) -> ()  [unwired: 2 in, 2 out]
            n173 = case shown="\"White Balance  **\"" w312 {
              tunnel: w311 -> [w318 w327 w336 w345 w354 _ w360]
              tunnel: w310 -> [w316 w324 w333 w342 w351 _ _]
              frame "Size  **" {
                n174 = Index Array(array=w316) -> (element=w315:cluster{string[]})  [unwired: 1 in]
                n175 = call <vilib>:"NT Read String.vi"("Name"=w318) -> ("String"=w317:string)  [unwired: 9 in, 1 out]
                n176 = Unbundle(w315) -> (w313:string[])
                n177 = Match First String(2:w313, 3:w317) -> (0:w314:i32)  [unwired: 1 out]
                n178 = property on="Ring" class="Ring (strict)"("Value"=w314, "Strings []"=w313) -> ()  [unwired: 2 in, 2 out]
                n179 = property on="Ring" class="Ring (strict)"("Visible"=TRUE) -> ()  [unwired: 2 in, 2 out]
                n180 = property on="Slider" class="Slide (strict)"("Visible"=FALSE) -> ()  [unwired: 2 in, 2 out]
              }
              frame "White Balance  **" {
                n181 = Index Array(array=w324, index=1) -> (element=w325:cluster{string[]})
                n182 = call <vilib>:"NT Read String.vi"("Name"=w327) -> ("String"=w326:string)  [unwired: 9 in, 1 out]
                n183 = Unbundle(w325) -> (w322:string[])
                n184 = Match First String(2:w322, 3:w326) -> (0:w321:i32)  [unwired: 1 out]
                n185 = property on="Ring" class="Ring (strict)"("Value"=w321, "Strings []"=w322) -> ()  [unwired: 2 in, 2 out]
                n186 = property on="Ring" class="Ring (strict)"("Visible"=TRUE) -> ()  [unwired: 2 in, 2 out]
                n187 = property on="Slider" class="Slide (strict)"("Visible"=FALSE) -> ()  [unwired: 2 in, 2 out]
              }
              frame "Exposure  **" {
                n188 = Index Array(array=w333, index=2) -> (element=w334:cluster{string[]})
                n189 = call <vilib>:"NT Read String.vi"("Name"=w336) -> ("String"=w335:string)  [unwired: 9 in, 1 out]
                n190 = Unbundle(w334) -> (w330:string[])
                n191 = Match First String(2:w330, 3:w335) -> (0:w331:i32)  [unwired: 1 out]
                n192 = property on="Ring" class="Ring (strict)"("Value"=w331, "Strings []"=w330) -> ()  [unwired: 2 in, 2 out]
                n193 = property on="Ring" class="Ring (strict)"("Visible"=TRUE) -> ()  [unwired: 2 in, 2 out]
                n194 = property on="Slider" class="Slide (strict)"("Visible"=FALSE) -> ()  [unwired: 2 in, 2 out]
              }
              frame "Exposure Priority  **" {
                n195 = Index Array(array=w342, index=3) -> (element=w343:cluster{string[]})
                n196 = call <vilib>:"NT Read String.vi"("Name"=w345) -> ("String"=w344:string)  [unwired: 9 in, 1 out]
                n197 = Unbundle(w343) -> (w339:string[])
                n198 = Match First String(2:w339, 3:w344) -> (0:w340:i32)  [unwired: 1 out]
                n199 = property on="Ring" class="Ring (strict)"("Value"=w340, "Strings []"=w339) -> ()  [unwired: 2 in, 2 out]
                n200 = property on="Ring" class="Ring (strict)"("Visible"=TRUE) -> ()  [unwired: 2 in, 2 out]
                n201 = property on="Slider" class="Slide (strict)"("Visible"=FALSE) -> ()  [unwired: 2 in, 2 out]
              }
              frame "Color Enable  **" {
                n202 = Index Array(array=w351, index=4) -> (element=w352:cluster{string[]})
                n203 = call <vilib>:"NT Read String.vi"("Name"=w354) -> ("String"=w353:string)  [unwired: 9 in, 1 out]
                n204 = Unbundle(w352) -> (w348:string[])
                n205 = Match First String(2:w348, 3:w353) -> (0:w349:i32)  [unwired: 1 out]
                n206 = property on="Ring" class="Ring (strict)"("Value"=w349, "Strings []"=w348) -> ()  [unwired: 2 in, 2 out]
                n207 = property on="Ring" class="Ring (strict)"("Visible"=TRUE) -> ()  [unwired: 2 in, 2 out]
                n208 = property on="Slider" class="Slide (strict)"("Visible"=FALSE) -> ()  [unwired: 2 in, 2 out]
              }
              frame Default {
                n209 = property on="Ring" class="Ring (strict)"("Visible"=FALSE) -> ()  [unwired: 2 in, 2 out]
                n210 = property on="Slider" class="Slide (strict)"("Visible"=FALSE) -> ()  [unwired: 2 in, 2 out]
              }
              frame "Brightness  **", "Color Level  **", "Compression  **", "FPS  **", "Sharpness  **" {
                n211 = call <vilib>:"NT Read Number.vi"("Name"=w360) -> ("Numeric"=w359:dbl)  [unwired: 9 in, 1 out]
                n212 = local write "Slider"(w359) -> ()
                n213 = property on="Slider" class="Slide (strict)"("Visible"=TRUE, "Scale.Maximum"=100.0 ("Scale.Range:Maximum")) -> ()  [unwired: 2 in, 2 out]
                n214 = property on="Ring" class="Ring (strict)"("Visible"=FALSE) -> ()  [unwired: 2 in, 2 out]
              }
            }
          }
        }
        n215 = property on="Progress" class="Clust (strict)"("Visible"=FALSE) -> ()  [unwired: 2 in, 2 out]
      }
      event "Test Name": Mouse Enter {
        # "Populate the ring with the list of tests"
        n216 = event-data() -> ()  [unwired: 1 in, 1 out]
        n217 = call <vilib>:"NT Read String Array.vi"("Name"="TestMode/TestList") -> ("String Array"=w367:string[])  [unwired: 9 in, 1 out]
        n218 = Build Array (concatenate)("Select the test to run...", w367) -> (w366:string[])
        n219 = property on="Test Name" class="Ring (strict)"("Strings []"=w366) -> ()  [unwired: 2 in, 2 out]
      }
      event "Test Name": Value Change {
        w369 = FALSE ("Visible")
        # "Tell the robot the test name to run"
        n220 = event-data() -> ("NewVal"=w373:u16)  [unwired: 1 in]
        n221 = property on="Test Name" class="Ring (strict)"() -> ("Strings []"=w374:string[])  [unwired: 2 in, 2 out]
        n222 = local write "Progress"(T4 {"Test Progress"=0, "Test Progress Text"=""} ("Progress")) -> ()
        n223 = Index Array(array=w374, index=w373) -> (element=w372:string)
        n224 = call <vilib>:"NT Write String.vi"("String"=w372, "Name"="TestMode/TestName") -> ()  [unwired: 9 in, 1 out]
        n225 = property on="Progress" class="Clust (strict)"("Visible"=TRUE) -> ()  [unwired: 2 in, 2 out]
        n226 = property on="Motor" class="Clust (strict)"("Visible"=w369) -> ()  [unwired: 2 in, 2 out]
        n227 = property on="Slider" class="Slide (strict)"("Visible"=w369) -> ()  [unwired: 2 in, 2 out]
        n228 = property on="On/Off" class="Bool (strict)"("Visible"=w369) -> ()  [unwired: 2 in, 2 out]
        n229 = property on="Rev/Fwd" class="Clust (strict)"("Visible"=w369) -> ()  [unwired: 2 in, 2 out]
        n230 = property on="Ring" class="Ring (strict)"("Visible"=w369) -> ()  [unwired: 2 in, 2 out]
      }
      event "Listbox": Double Click {
        n231 = event-data() -> ("PlatMods.Shift"=w377:bool, "Row"=w379:i32)  [unwired: 1 in]
        n232 = case shown="False" w377 {
          tunnel: w379 -> [w383 _]
          tunnel: 1 -> [w382 _]
          frame False {
            n233 = property on="Listbox" class="LstBox (strict)"() -> ("Item Symbols"=w381:i32[])  [unwired: 2 in, 2 out]
            n234 = Replace Array Subset(array=w381, new element=w382, index=w383) -> (w380:i32[])
            n235 = property on="Listbox" class="LstBox (strict)"("Item Symbols"=w380) -> ()  [unwired: 2 in, 2 out]
          }
          frame True {
            w384 = 0 ("Top Row")
            n236 = property on="Listbox" class="LstBox (strict)"() -> ("Number of Rows"=w386:u32)  [unwired: 2 in, 2 out]
            n237 = Initialize Array(0, w386) -> (w385:i32[])
            n238 = property on="Listbox" class="LstBox (strict)"("Top Row"=w384, "Value"=w384, "Item Symbols"=w385) -> ()  [unwired: 2 in, 2 out]
          }
        }
      }
      event "Listbox": Key Down {
        n239 = event-data() -> ("VKey"=w390:T19)  [unwired: 1 in]
        n240 = case shown="\"Left\", \"Right\"" w390 {
          selector: w390 -> [w395 _]
          tunnel: eventvkey."Left" ("VKey") -> [w393 _]
          frame "Left", "Right" {
            n241 = Equal?(x=w393, y=w395) -> (x = y?=w394:bool)
            n242 = Select(t=0, s=w394, f=1) -> (s? t:f=w396:i32)
            n243 = property on="Listbox" class="LstBox (strict)"() -> ("Item Symbols"=w399:i32[])  [unwired: 2 in, 2 out]
            n244 = Replace Array Subset(array=w399, new element=w396, index="Listbox") -> (w398:i32[])
            n245 = property on="Listbox" class="LstBox (strict)"("Item Symbols"=w398) -> ()  [unwired: 2 in, 2 out]
          }
          frame Default {
          }
        }
      }
      event "DB Camera Config": Value Change {
        n246 = event-data() -> ("NewVal"=w403:bool)  [unwired: 1 in]
        n247 = case shown="False" w403 {
          tunnel: w402 -> [w412 _]
          tunnel: [w405 w423] -> w401
          tunnel: w400 -> [w404 w423]
          frame False {
            w419 = "Camera"
            w422 = FALSE ("Visible")
            n248 = local read "Camera Settings"() -> (w411:T1)
            n249 = Index Array(array=w412) -> (element=w415:cluster{string[]})  [unwired: 1 in]
            n250 = Unbundle(w411) -> ("Frate Rate"=w410:i32, "Compression"=w409:i32, "Size"=w413:u16)
            n251 = Unbundle(w415) -> (w414:string[])
            n252 = Index Array(array=w414, index=w413) -> (element=w408:string)
            n253 = call-poly <vilib>:"Write Key.vi"("section"=w419, "value"=w408, "key"="Size", "refnum"=w404) -> ("refnum out"=w421:T18)  [unwired: 2 in, 5 out]
            n254 = call-poly <vilib>:"Write Key.vi"("section"=w419, "value"=w410, "key"="FrameRate", "refnum"=w421) -> ("refnum out"=w420:T18)  [unwired: 1 in, 6 out]
            n255 = property on="Camera Settings" class="Clust (strict)"("Visible"=w422) -> ()  [unwired: 2 in, 2 out]
            n256 = local write "DB Camera Config"(w422) -> ()
            n257 = call-poly <vilib>:"Write Key.vi"("section"=w419, "value"=w409, "key"="Compression", "refnum"=w420) -> ("refnum out"=w406:T18)  [unwired: 1 in, 6 out]
            n258 = call <vilib>:"Close Config Data.vi"("refnum"=w406) -> ("file path"=w407:path)  [unwired: 2 in, 8 out]
            n259 = call <vilib>:"Open Config Data.vi"("configuration file path"=w407) -> ("refnum"=w405:T18)  [unwired: 8 in, 2 out]
          }
          frame True {
            n260 = property on="Camera Settings" class="Clust (strict)"("Visible"=TRUE) -> ()  [unwired: 2 in, 2 out]
          }
        }
      }
      event "Camera Settings": Value Change {
        n261 = event-data() -> ("NewVal"=w436:T1)  [unwired: 1 in]
        n262 = Index Array(array=w432) -> (element=w431:cluster{string[]})  [unwired: 1 in]
        n263 = Unbundle(w436) -> ("Frate Rate"=w427:i32, "Compression"=w426:i32, "Size"=w429:u16)
        n264 = Unbundle(w431) -> (w430:string[])
        n265 = Index Array(array=w430, index=w429) -> (element=w428:string)
        n266 = Format Into String(format string="%s   %dfps   %d%%", w428, w427, w426) -> (resulting string=w433:string)  [unwired: 2 in, 1 out]
        n267 = Build Array(w433) -> (w434:string[])
        n268 = property on="DB Camera Config" class="Bool (strict)"("Strings [4]"=w434) -> ()  [unwired: 2 in, 2 out]
      }
      event "Motor.Enable": Value Change {
        n269 = event-data() -> ("NewVal"=w442:bool)  [unwired: 1 in]
        n270 = Unbundle("Motor") -> ("Value"=w441:dbl)  [unwired: 1 out]
        n271 = Select(t=w441, s=w442, f=0.0) -> (s? t:f=w439:dbl)
        n272 = call <vilib>:"NT Write Number.vi"("Numeric"=w439, "Name"=w438) -> ()  [unwired: 9 in, 1 out]
      }
      event "Slider": Value Change {
        n273 = event-data() -> ("NewVal"=w445:dbl)  [unwired: 1 in]
        n274 = call <vilib>:"NT Write Number.vi"("Numeric"=w445, "Name"=w446) -> ()  [unwired: 9 in, 1 out]
      }
      event "On/Off": Value Change {
        n275 = event-data() -> ("NewVal"=w450:bool)  [unwired: 1 in]
        n276 = Boolean To (0,1)(Boolean=w450) -> (0, 1=w449:i16)
        n277 = call <vilib>:"NT Write Number.vi"("Numeric"=w449, "Name"=w448) -> ()  [unwired: 9 in, 1 out]
      }
      event "Rev/Fwd": Value Change {
        n278 = event-data() -> ("NewVal.Forward"=w458:bool, "NewVal.Reverse"=w457:bool)  [unwired: 1 in]
        n279 = Boolean To (0,1)(Boolean=w458) -> (0, 1=w454:i16)
        n280 = Boolean To (0,1)(Boolean=w457) -> (0, 1=w456:i16)
        n281 = Negate(x=w456) -> (-x=w455:i16)
        n282 = Add(x=w454, y=w455) -> (x+y=w453:i16)
        n283 = call <vilib>:"NT Write Number.vi"("Numeric"=w453, "Name"=w452) -> ()  [unwired: 9 in, 1 out]
      }
      event "Ring": Value Change {
        n284 = event-data() -> ("NewVal"=w462:u16)  [unwired: 1 in]
        n285 = property on="Ring" class="Ring (strict)"() -> ("Strings []"=w463:string[])  [unwired: 2 in, 2 out]
        n286 = Index Array(array=w463, index=w462) -> (element=w461:string)
        n287 = call <vilib>:"NT Write String.vi"("String"=w461, "Name"=w460) -> ()  [unwired: 9 in, 1 out]
      }
    }
  }
  n288 = Index Array(array=w16) -> (element=w17:cluster{string[]})  [unwired: 1 in]
  n289 = Unbundle(w17) -> (w15:string[])
  n290 = Match First String(2:w15, 3:w14) -> (0:w13:i32)  [unwired: 1 out]
  n291 = Bundle("value"=w19, "value"=w18, "index"=w13) -> (w7:cluster{"value":i32, "value":i32, "index":i32})  [unwired: 1 out]
  n292 = property on="On/Off" class="Bool (strict)"("Visible"=w30) -> ()  [unwired: 2 in, 2 out]
  n293 = property on="Motor" class="Clust (strict)"("Visible"=w30) -> ()  [unwired: 2 in, 2 out]
  n294 = property on="Progress" class="Clust (strict)"("Visible"=w30) -> ()  [unwired: 2 in, 2 out]
  n295 = property on="Ring" class="Ring (strict)"("Visible"=w30) -> ()  [unwired: 2 in, 2 out]
  n296 = property on="Camera Settings" class="Clust (strict)"("Val(Sgnl)"=w7) -> ()  [unwired: 2 in, 2 out]
  n297 = property on="Rev/Fwd" class="Clust (strict)"("Visible"=w30) -> ()  [unwired: 2 in, 2 out]
  n298 = property on="Camera Settings" class="Clust (strict)"("Visible"=w30) -> ()  [unwired: 2 in, 2 out]
  n299 = local write "DB Camera Config"(w30) -> ()
